vi "PH_HamamatsuCamera.evt call SetTriggerParameter.vi"(0 "i ref in":refnum<vi>, 2 "Instance":string, 3 "Trigger Parameters":T1={"Mode"=1, "Polarity"=1, "Times"=1, "Delay"=0.0} {"Polarity" items=["Negative"=1, "Positive"=2]; "Mode" items=["Internal"=1, "External Edge"=2, "External Level"=4, "Software"=32, "Fast Repetition"=64, "TDI"=128, "Trigger Start"=512, "Sync Readout"=1024]}, 5 "error in (no error)":errorcluster) -> (14 "i ref out":refnum<vi>, 19 "error out":errorcluster)   [LabVIEW 2014, in "PH_HamamatsuCamera.lvlib"]
doc: "This VI sends a simple call for SetTriggerType."
uses:
  PH_HamamatsuCamera.lvlib
  PH_HamamatsuCamera.Trigger Parameter.ctl
  CS_Core/CSSystem/CoreLib/CoreLib.double 2 byte array.vi
  CS_Core/CSSystem/CoreLib/CoreLib.int 2 byte array.vi
  CS_Core/CSSystem/CoreLib/CoreLib.lvlib
  CS_Core/BaseProcess/BaseProcess.lvlib
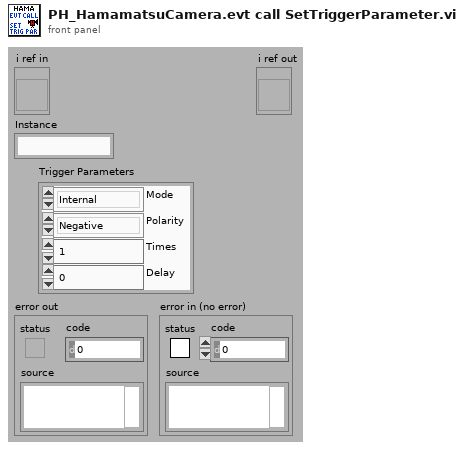
[diagram p1: front panel]
types:
  T1 = typedef "PH_HamamatsuCamera.lvlib/PH_HamamatsuCamera.Trigger Parameter.ctl" = cluster{"Mode":u32, "Polarity":u32, "Times":u32, "Delay":dbl}
  T2 = typedef "CoreDefs.rawDataType.ctl" = i8[]
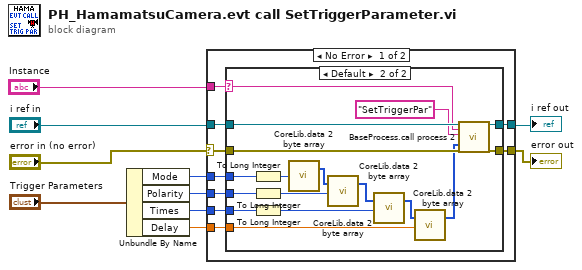
[diagram p0: block diagram]
diagram:
  n1 = Unbundle By Name("Trigger Parameters") -> ("Mode"=w4:u32, "Polarity"=w3:u32, "Times"=w2:u32, "Delay"=w1:dbl)
  n2 = case shown="No Error" "error in (no error)" {
    selector: "error in (no error)" -> [w15 w39]
    tunnel: [w19 w40] -> w9
    tunnel: [w18 w39] -> w8
    tunnel: "i ref in" -> [w17 w40]
    tunnel: "Instance" -> [w14 _]
    tunnel: w4 -> [w16 _]
    tunnel: w3 -> [w13 _]
    tunnel: w2 -> [w12 _]
    tunnel: w1 -> [w11 _]
    frame No Error {
      n3 = case shown="Default" w14 {
        selector: w14 -> [_ w24]
        tunnel: [w21 w38] -> w19
        tunnel: [w20 w37] -> w18
        tunnel: w17 -> [w21 w36]
        tunnel: w16 -> [_ w33]
        tunnel: w15 -> [w20 w32]
        tunnel: w13 -> [_ w31]
        tunnel: w12 -> [_ w30]
        tunnel: w11 -> [_ w29]
        frame "N/A" {
        }
        frame Default {
          n4 = To Long Integer(number=w33) -> (32bit integer=w34:i32)
          n5 = To Long Integer(number=w31) -> (32bit integer=w23:i32)
          n6 = To Long Integer(number=w30) -> (32bit integer=w22:i32)
          n7 = call-poly "CoreLib.data 2 byte array.vi"("i32"=w34) -> ("byteArray out"=w27:T2)  [unwired: 18 in]
          n8 = call-poly "CoreLib.data 2 byte array.vi"("byteArray"=w27, "i32"=w23) -> ("byteArray out"=w26:T2)  [unwired: 17 in]
          n9 = call-poly "CoreLib.data 2 byte array.vi"("byteArray"=w26, "i32"=w22) -> ("byteArray out"=w25:T2)  [unwired: 17 in]
          n10 = call-poly "CoreLib.data 2 byte array.vi"("byteArray"=w25, "f64"=w29) -> ("byteArray out"=w28:T2)  [unwired: 17 in]
          n11 = call "BaseProcess.call process 2.vi"("i ref in"=w36, "Object"=w24, "Selector"="SetTriggerPar", "Data"=w28, "error in (no error)"=w32) -> ("i ref out"=w38:refnum<vi>, "error out"=w37:errorcluster)  [unwired: 13 in]
        }
      }
    }
    frame Error {
    }
  }
  "error out" <- w8
  "i ref out" <- w9
